vi "LL_Atmion_test.vi"() -> ()   [LabVIEW 2014]
uses:
  <vilib>/Instr/_visa.llb/VISA Configure Serial Port (Instr).vi
  <userlib>/Nanonis Prog Interface V5/Nanonis Prog Interface.lvlib
panel:
  in  "stop":bool
  out "concatenated string":string
  out "Serial Settings:Number of Bytes at Serial Port":u32
  in  "milliseconds to wait":u32
  in  "baud rate (9600)":u32=9600
  in  "termination char\n(0xA = '\\n' = LF)":u8=10 format="%.0x"
  in  "write buffer":string
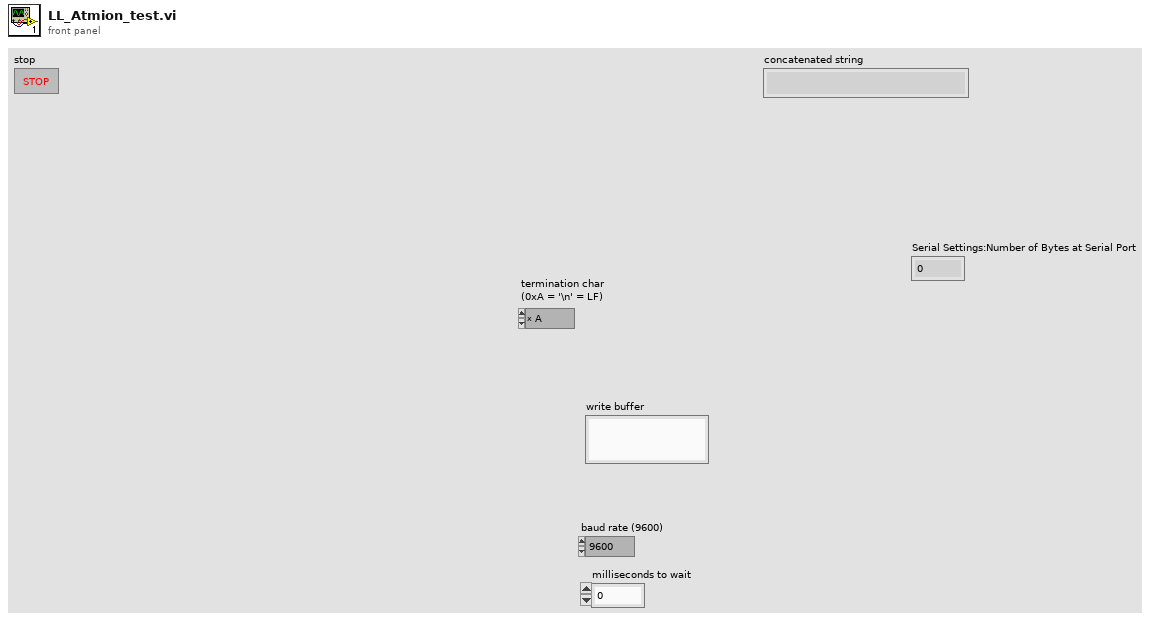
[diagram p1: front panel]
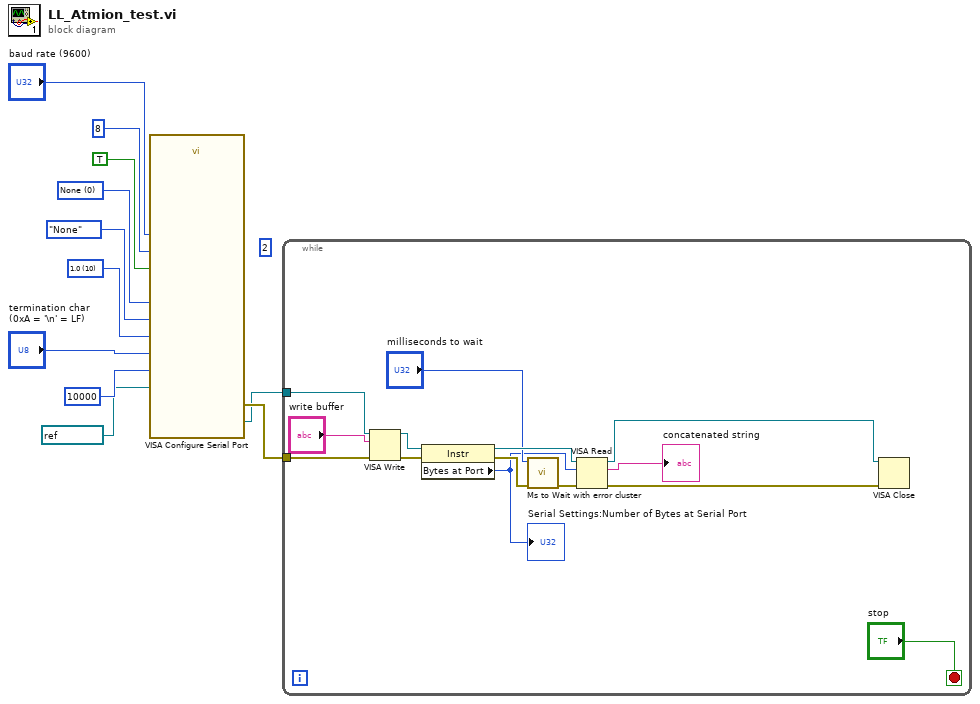
[diagram p0: block diagram]
diagram:
  (unwired) 2
  w4 = u16 0 items=["None", "XON/XOFF", "RTS/CTS", "XON/XOFF & RTS/CTS", "DTR/DSR", "XON/XOFF & DTR/DSR"] ("flow control (0:none)")
  w5 = u16 10 items=["1.0"=10, "1.5"=15, "2.0"=20] ("stop bits (10: 1 bit)")
  n1 = call-poly "VISA Configure Serial Port"("VISA resource name"=refnum<visa-resource-name> "COM7", "timeout (10sec)"=u32 10000, "termination char\n(0xA = '\\n' = LF)"="termination char\n(0xA = '\\n' = LF)", "Enable Termination\nChar (T)"=TRUE ("Enable Termination\nChar (T)"), "baud rate (9600)"="baud rate (9600)", "data bits (8)"=u16 8, "parity (0:none)"=enum16{"None", "Odd", "Even", "Mark", "Space"}."None", "stop bits (10: 1 bit)"=w5, "flow control (0:none)"=w4) -> ("VISA resource name out"=w1:refnum<visa-resource-name>, "error out"=w3:errorcluster)  [unwired: 5 in]
  n2 = while {
    tunnel: w3 -> [w23]
    tunnel: w1 -> [w22]
    stop <- "stop" stop-if-true
    n3 = VISA Write(VISA resource name=w22, write buffer="write buffer", error in (no error)=w23) -> (VISA resource name out=w20:refnum<visa-resource-name>, error out=w18:errorcluster)  [unwired: 1 out]
    n4 = property class="Instr"(reference=w20, error in=w18) -> (reference out=w21:refnum<visa-resource-name>, error out=w17:errorcluster, "Bytes at Port"=w14:u32)
    "Serial Settings:Number of Bytes at Serial Port" <- w14
    n5 = call <userlib>:"Ms to Wait with error cluster.vi"("error in (no error)"=w17, "milliseconds to wait"="milliseconds to wait") -> ("error out"=w16:errorcluster)  [unwired: 4 in, 1 out]
    n6 = VISA Read(VISA resource name=w21, byte count=w14, error in (no error)=w16) -> (VISA resource name out=w25:refnum<visa-resource-name>, read buffer=→"concatenated string":string, error out=w24:errorcluster)  [unwired: 1 out]
    n7 = VISA Close(VISA resource name=w25, error in (no error)=w24) -> ()  [unwired: 1 out]
  }
